vi "Button_toggle_5_input.vi"(0 "in 1":bool, 5 "in 2":bool, 7 "in3":bool, 9 "in 4":bool, 11 "in 5":bool) -> (4 "Out 1":bool, 6 "Out 2":bool, 8 "Out3":bool, 10 "Out 4":bool, 15 "out 5":bool)   [LabVIEW 2020]
panel:
  out "toggle if other 5":bool
  out "toggle if other 4":bool
  out "toggle if other 3":bool
  out "toggle if other 2":bool
  out "toggle if other":bool
  out "one press\n 5":bool
  out "one press\n 4":bool
  out "one press\n 3":bool
  out "one press\n 2":bool
  out "one press":bool
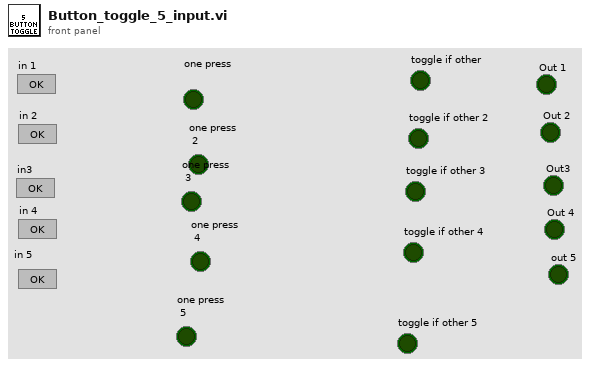
[diagram p1: front panel]
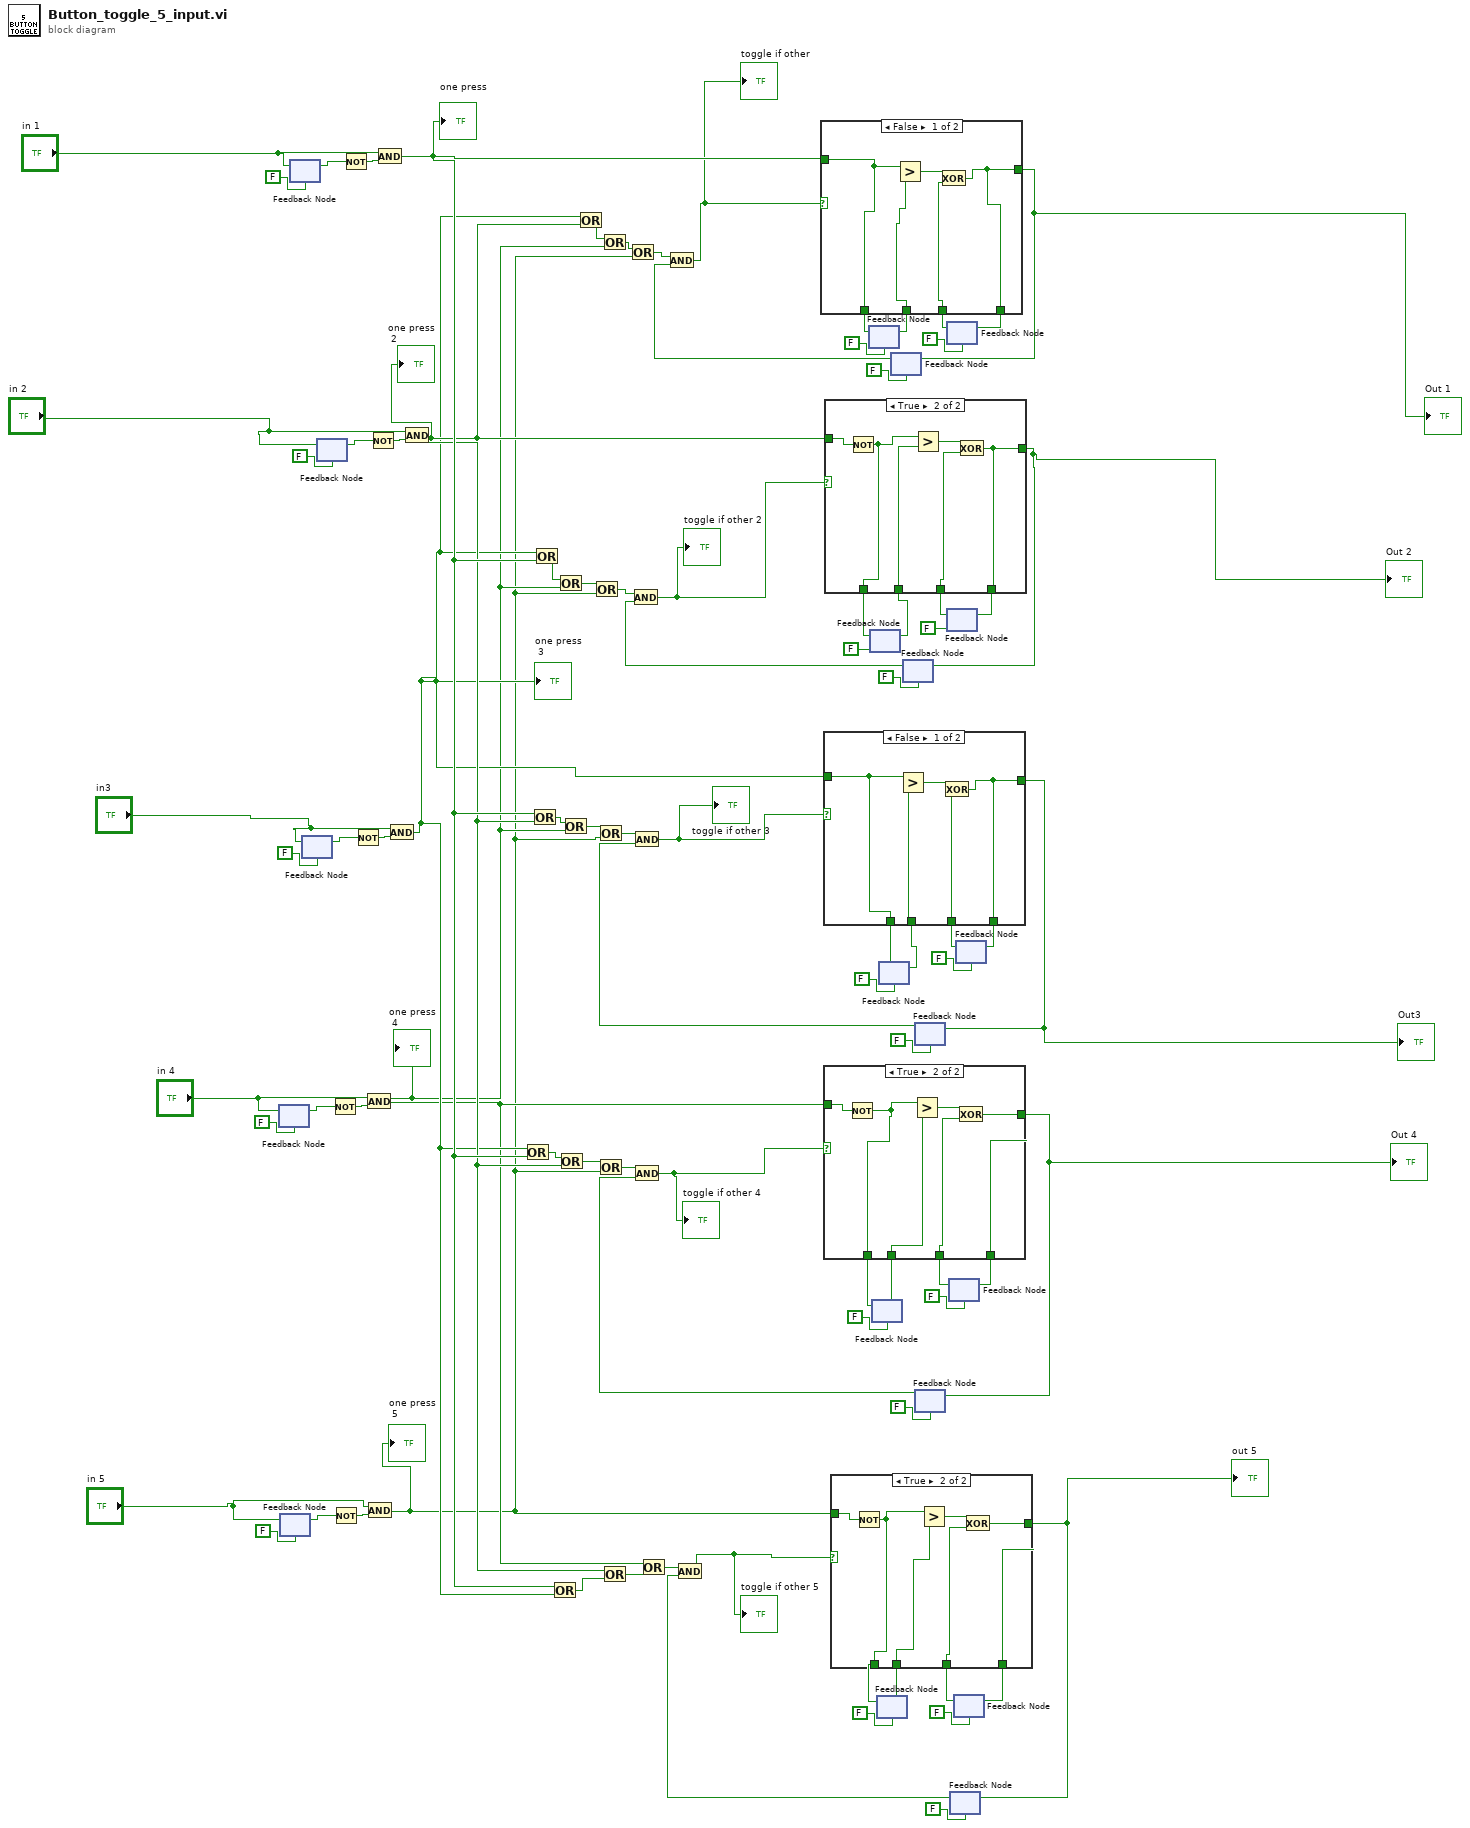
[diagram p0: block diagram]
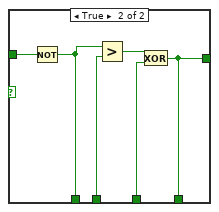
[diagram p2: hidden frame]
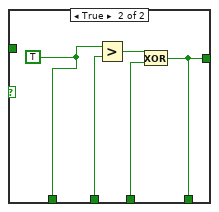
[diagram p3: hidden frame]
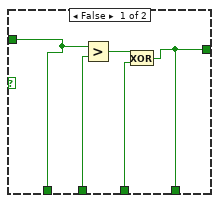
[diagram p4: hidden frame]
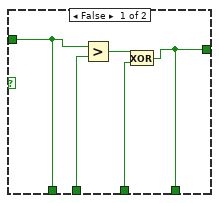
[diagram p5: hidden frame]
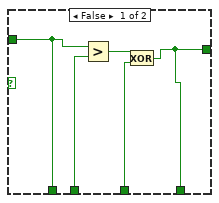
[diagram p6: hidden frame]
diagram:
  n1 = feedback #1(FALSE) -> (w47:bool)
  n2 = feedback-in #1("in 4") -> ()
  n3 = feedback #2(FALSE) -> (w43:bool)
  n4 = feedback-in #2("in 5") -> ()
  n5 = feedback #3(FALSE) -> (w51:bool)
  n6 = feedback-in #3("in 1") -> ()
  n7 = feedback #4(FALSE) -> (w79:bool)
  n8 = feedback-in #4("in3") -> ()
  n9 = feedback #5(FALSE) -> (w48:bool)
  n10 = feedback-in #5("in 2") -> ()
  n11 = Not(x=w47) -> (.not. x?=w46:bool)
  n12 = Not(x=w43) -> (.not. x?=w44:bool)
  n13 = Not(x=w51) -> (.not. x?=w50:bool)
  n14 = Not(x=w79) -> (.not. x?=w80:bool)
  n15 = And(x="in 4", y=w46) -> (x .and. y?=w37:bool)
  "one press\n 4" <- w37
  n16 = And(x="in 5", y=w44) -> (x .and. y?=w36:bool)
  "one press\n 5" <- w36
  n17 = Not(x=w48) -> (.not. x?=w49:bool)
  n18 = And(x="in 1", y=w50) -> (x .and. y?=w40:bool)
  "one press" <- w40
  n19 = And(x="in3", y=w80) -> (x .and. y?=w38:bool)
  "one press\n 3" <- w38
  n20 = And(x="in 2", y=w49) -> (x .and. y?=w39:bool)
  "one press\n 2" <- w39
  n21 = Or(x=w38, y=w40) -> (x .or. y?=w85:bool)
  n22 = Or(x=w40, y=w39) -> (x .or. y?=w86:bool)
  n23 = Or(x=w38, y=w40) -> (x .or. y?=w87:bool)
  n24 = Or(x=w40, y=w38) -> (x .or. y?=w84:bool)
  n25 = Or(x=w87, y=w37) -> (x .or. y?=w60:bool)
  n26 = Or(x=w85, y=w39) -> (x .or. y?=w57:bool)
  n27 = Or(x=w86, y=w37) -> (x .or. y?=w74:bool)
  n28 = Or(x=w38, y=w39) -> (x .or. y?=w88:bool)
  n29 = Or(x=w60, y=w36) -> (x .or. y?=w61:bool)
  n30 = Or(x=w74, y=w36) -> (x .or. y?=w76:bool)
  n31 = Or(x=w57, y=w36) -> (x .or. y?=w55:bool)
  n32 = Or(x=w88, y=w37) -> (x .or. y?=w65:bool)
  n33 = Or(x=w39, y=w84) -> (x .or. y?=w52:bool)
  n34 = Or(x=w65, y=w36) -> (x .or. y?=w64:bool)
  n35 = Or(x=w37, y=w52) -> (x .or. y?=w45:bool)
  n36 = feedback #6(FALSE) -> (w29:bool)
  n37 = feedback #7(FALSE) -> (w21:bool)
  n38 = feedback #8(FALSE) -> (w9:bool)
  n39 = feedback #9(FALSE) -> (w3:bool)
  n40 = feedback #10(FALSE) -> (w15:bool)
  n41 = feedback #11(FALSE) -> (w66:bool)
  n42 = And(x=w64, y=w66) -> (x .and. y?=w35:bool)
  "toggle if other" <- w35
  n43 = feedback #12(FALSE) -> (w62:bool)
  n44 = And(x=w61, y=w62) -> (x .and. y?=w34:bool)
  "toggle if other 2" <- w34
  n45 = feedback #13(FALSE) -> (w75:bool)
  n46 = And(x=w76, y=w75) -> (x .and. y?=w32:bool)
  "toggle if other 3" <- w32
  n47 = feedback #14(FALSE) -> (w56:bool)
  n48 = And(x=w55, y=w56) -> (x .and. y?=w33:bool)
  "toggle if other 4" <- w33
  n49 = feedback #15(FALSE) -> (w26:bool)
  n50 = case shown="False" w35 {
    tunnel: [w92 w96] -> w72
    tunnel: w40 -> [w94 _]
    tunnel: w29 -> [w93 w99]
    tunnel: [w94 w98] -> w28
    tunnel: w26 -> [w91 w97]
    tunnel: [w92 w96] -> w25
    frame False {
      n51 = Greater?(x=w94, y=w93) -> (0:w95:bool)
      n52 = Exclusive Or(1:w91, 2:w95) -> (0:w92:bool)
    }
    frame True {
      w98 = TRUE
      n53 = Greater?(x=w98, y=w99) -> (0:w100:bool)
      n54 = Exclusive Or(1:w97, 2:w100) -> (0:w96:bool)
    }
  }
  "Out 1" <- w72
  n55 = feedback-in #6(w28) -> ()
  n56 = feedback-in #11(w72) -> ()
  n57 = feedback-in #15(w25) -> ()
  n58 = feedback #16(FALSE) -> (w22:bool)
  n59 = case shown="True" w34 {
    tunnel: [w102 w109] -> w89
    tunnel: w39 -> [w101 w110]
    tunnel: w22 -> [w104 w106]
    tunnel: w21 -> [w103 w107]
    tunnel: [w102 w109] -> w20
    tunnel: [w101 w108] -> w19
    frame False {
      n60 = Greater?(x=w101, y=w103) -> (0:w105:bool)
      n61 = Exclusive Or(1:w104, 2:w105) -> (0:w102:bool)
    }
    frame True {
      n62 = Not(x=w110) -> (.not. x?=w108:bool)
      n63 = Greater?(x=w108, y=w107) -> (0:w111:bool)
      n64 = Exclusive Or(1:w106, 2:w111) -> (0:w109:bool)
    }
  }
  "Out 2" <- w89
  n65 = feedback-in #7(w19) -> ()
  n66 = feedback-in #12(w89) -> ()
  n67 = feedback-in #16(w20) -> ()
  n68 = feedback #17(FALSE) -> (w10:bool)
  n69 = case shown="True" w33 {
    tunnel: [w112 w117] -> w90
    tunnel: w37 -> [w113 w121]
    tunnel: w10 -> [w115 w118]
    tunnel: w9 -> [w114 w119]
    tunnel: [w113 w120] -> w8
    tunnel: [w112 w117] -> w7
    frame False {
      n70 = Greater?(x=w113, y=w114) -> (0:w116:bool)
      n71 = Exclusive Or(1:w115, 2:w116) -> (0:w112:bool)
    }
    frame True {
      n72 = Not(x=w121) -> (.not. x?=w120:bool)
      n73 = Greater?(x=w120, y=w119) -> (0:w122:bool)
      n74 = Exclusive Or(1:w118, 2:w122) -> (0:w117:bool)
    }
  }
  "Out 4" <- w90
  n75 = feedback-in #8(w8) -> ()
  n76 = feedback-in #14(w90) -> ()
  n77 = feedback-in #17(w7) -> ()
  n78 = feedback #18(FALSE) -> (w54:bool)
  n79 = And(x=w45, y=w54) -> (x .and. y?=w31:bool)
  "toggle if other 5" <- w31
  n80 = feedback #19(FALSE) -> (w4:bool)
  n81 = case shown="True" w31 {
    tunnel: [w123 w128] -> w53
    tunnel: w36 -> [w124 w132]
    tunnel: w4 -> [w126 w129]
    tunnel: w3 -> [w125 w130]
    tunnel: [w124 w131] -> w2
    tunnel: [w123 w128] -> w1
    frame False {
      n82 = Greater?(x=w124, y=w125) -> (0:w127:bool)
      n83 = Exclusive Or(1:w126, 2:w127) -> (0:w123:bool)
    }
    frame True {
      n84 = Not(x=w132) -> (.not. x?=w131:bool)
      n85 = Greater?(x=w131, y=w130) -> (0:w133:bool)
      n86 = Exclusive Or(1:w129, 2:w133) -> (0:w128:bool)
    }
  }
  "out 5" <- w53
  n87 = feedback-in #9(w2) -> ()
  n88 = feedback-in #18(w53) -> ()
  n89 = feedback-in #19(w1) -> ()
  n90 = feedback #20(FALSE) -> (w16:bool)
  n91 = case shown="False" w32 {
    tunnel: [w136 w140] -> w77
    tunnel: w38 -> [w137 w143]
    tunnel: w16 -> [w135 w142]
    tunnel: w15 -> [w134 w141]
    tunnel: [w136 w140] -> w14
    tunnel: [w137 w139] -> w13
    frame False {
      n92 = Greater?(x=w137, y=w134) -> (0:w138:bool)
      n93 = Exclusive Or(1:w135, 2:w138) -> (0:w136:bool)
    }
    frame True {
      n94 = Not(x=w143) -> (.not. x?=w139:bool)
      n95 = Greater?(x=w139, y=w141) -> (0:w144:bool)
      n96 = Exclusive Or(1:w142, 2:w144) -> (0:w140:bool)
    }
  }
  "Out3" <- w77
  n97 = feedback-in #10(w13) -> ()
  n98 = feedback-in #13(w77) -> ()
  n99 = feedback-in #20(w14) -> ()
